vi "Prog9.vi"() -> ()   [LabVIEW 2021]
panel:
  out "x = y?":bool
  out "length":i32
  out "string 2":string
  out "string":string
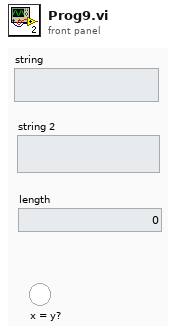
[diagram p1: front panel]
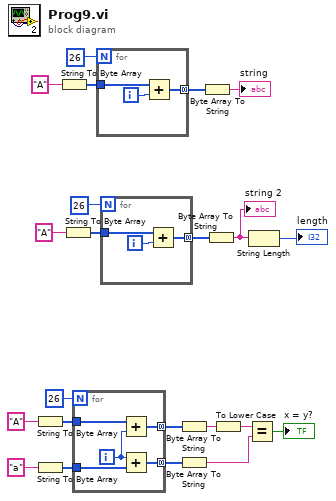
[diagram p0: block diagram]
diagram:
  n1 = String To Byte Array(string="A") -> (unsigned byte array=w10:u8[])
  n2 = String To Byte Array(string="a") -> (unsigned byte array=w7:u8[])
  n3 = String To Byte Array(string="A") -> (unsigned byte array=w21:u8[])
  n4 = String To Byte Array(string="A") -> (unsigned byte array=w17:u8[])
  n5 = for {
    N: 26 -> [_]
    tunnel: w10 -> [w27]
    tunnel: [w26] -> w9 mode=concatenating
    tunnel: w7 -> [w24]
    tunnel: [w23] -> w6 mode=concatenating
    i -> [w25]
    n6 = Add(x=w27, y=w25) -> (x+y=w26:i32[])
    n7 = Add(x=w25, y=w24) -> (x+y=w23:i32[])
  }
  n8 = for {
    N: 26 -> [_]
    tunnel: w21 -> [w29]
    tunnel: [w28] -> w20 mode=concatenating
    i -> [w30]
    n9 = Add(x=w29, y=w30) -> (x+y=w28:i32[])
  }
  n10 = for {
    N: 26 -> [_]
    tunnel: w17 -> [w32]
    tunnel: [w31] -> w16 mode=concatenating
    i -> [w33]
    n11 = Add(x=w32, y=w33) -> (x+y=w31:i32[])
  }
  n12 = Byte Array To String(unsigned byte array=w9) -> (string=w5:string)
  n13 = Byte Array To String(unsigned byte array=w6) -> (string=w3:string)
  n14 = Byte Array To String(unsigned byte array=w20) -> (string=→"string":string)
  n15 = Byte Array To String(unsigned byte array=w16) -> (string=w13:string)
  "string 2" <- w13
  n16 = To Lower Case(string=w5) -> (all lower case string=w4:string)
  n17 = Equal?(x=w4, y=w3) -> (x = y?=→"x = y?":bool)
  n18 = String Length(string=w13) -> (length=→"length":i32)
